vi "Actor Core.vi"(8 "error in":errorcluster, 11 "Instrument Finder in":refnum<class "Instrument Finder.lvclass">) -> (0 "error out":errorcluster, 3 "Actor out":refnum<class "Actor.lvclass">)   [LabVIEW 2014, in "SetUp VIs.lvlib" / "Instrument Finder.lvclass"]
doc: "(<B>Filename</B>: Actor Framework.lvlib:Actor.lvclass:Actor Core.vi)\n\nReceives messages to the actor, reacts to them, and initiates any error handling that may shut the actor down.\n\nDescendant classes may override this VI to append parallel tasks for the actor to complete while it handles messages. Overrides use the Call Parent Method node."
uses:
  Instrument Finder.lvclass
  <vilib>/ActorFramework/Actor/Actor.lvclass
  Controls/Instrument ID Object.ctl
  Generic Instrument/Generic Instrument.lvclass
  <vilib>/Instr/_visa.llb/VISA Find Search Mode.ctl
  <vilib>/ActorFramework/Actor/Actor.lvclass/Actor.ctl
  <vilib>/ActorFramework/Message Enqueuer/Message Enqueuer.lvclass/Message Enqueuer.ctl
  <vilib>/Utility/error.llb/DialogType.ctl
  <vilib>/ActorFramework/Report Error Msg/Report Error Msg.lvclass/Report Error Msg.ctl
  <vilib>/ActorFramework/Message Enqueuer/Message Priority.ctl
  Controller Messages/Write Instrument finder Done boolean to Ref Msg/Write Instrument finder Done boolean to Ref Msg.lvclass/Write Instrument finder Done boolean to Ref Msg.ctl
  <vilib>/ActorFramework/Stop Msg/Stop Msg.lvclass/Stop Msg.ctl
  Controller Messages/Write array of Instrument value to Ref Msg/Write array of Instrument value to Ref Msg.lvclass/Write array of Instrument value to Ref Msg.ctl
  <vilib>/ActorFramework/Message Enqueuer/Enqueue.vi
  <vilib>/ActorFramework/Message Enqueuer/Init from Existing Queue.vi
  <vilib>/ActorFramework/Message Enqueuer/Enqueue Critical.vi
  <vilib>/ActorFramework/Message Priority Queue/Priority Enqueue.vi
  <vilib>/ActorFramework/Report Error Msg/Report Error Msg.lvclass
  <vilib>/ActorFramework/Message Enqueuer/Message Enqueuer.lvclass
  Controller Messages/Write Instrument finder Done boolean to Ref Msg/Write Instrument finder Done boolean to Ref Msg.lvclass
  <vilib>/ActorFramework/Stop Msg/Stop Msg.lvclass
  Controller Messages/Write array of Instrument value to Ref Msg/Write array of Instrument value to Ref Msg.lvclass
  Subpanel Insertion/Subpanel Inserter.lvclass
  SetUp VIs.lvlib
panel:
  out "NaN/Path/Refnum?":bool
  out "done?":bool
  in  "Confirm":bool
  out "deleted portion 2":refnum<class "Generic Instrument.lvclass">
  out "Array":refnum<class "Generic Instrument.lvclass">[](array[class])
  out "error out 2":errorcluster
  out "deleted portion":T1
  out "# of time":i32
  out "selected instruments":T1[](array[typedef])
  out "index of element":i32
  out "data":T1
  out "find list":string[](array[string])
  out "i":i32
  out "Numeric Control":i32
  out "# of Instruments Found":i32
  in  "List of Instruments":T1[](array[typedef])
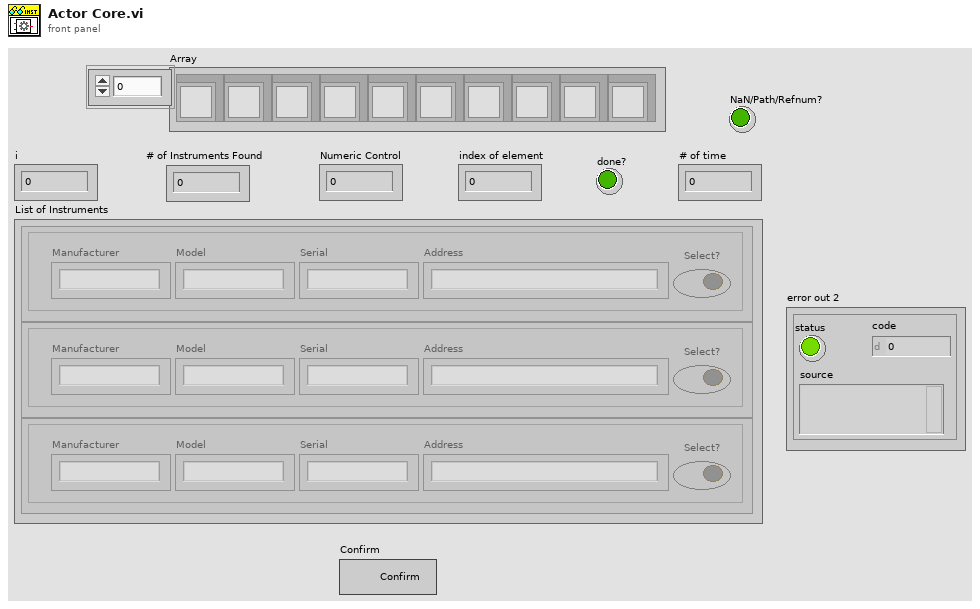
[diagram p1: front panel]
types:
  T1 = typedef "Instrument ID Object.ctl" = cluster{"Manufacturer":string, "Model":string, "Serial":string, "Address":string, "Select?":bool}
  T2 = cluster{"Manufacturer":string, "Model":string, "Serial":string, "Address":string, "Boolean":bool}[]
  T3 = typedef "VISA Find Search Mode.ctl" = u32
  T4 = typedef "DialogType.ctl" = u16
  T5 = typedef "Actor Framework.lvlib/Message Enqueuer.lvclass/Message Priority.ctl" = enum16{"Low", "Normal", "High"}
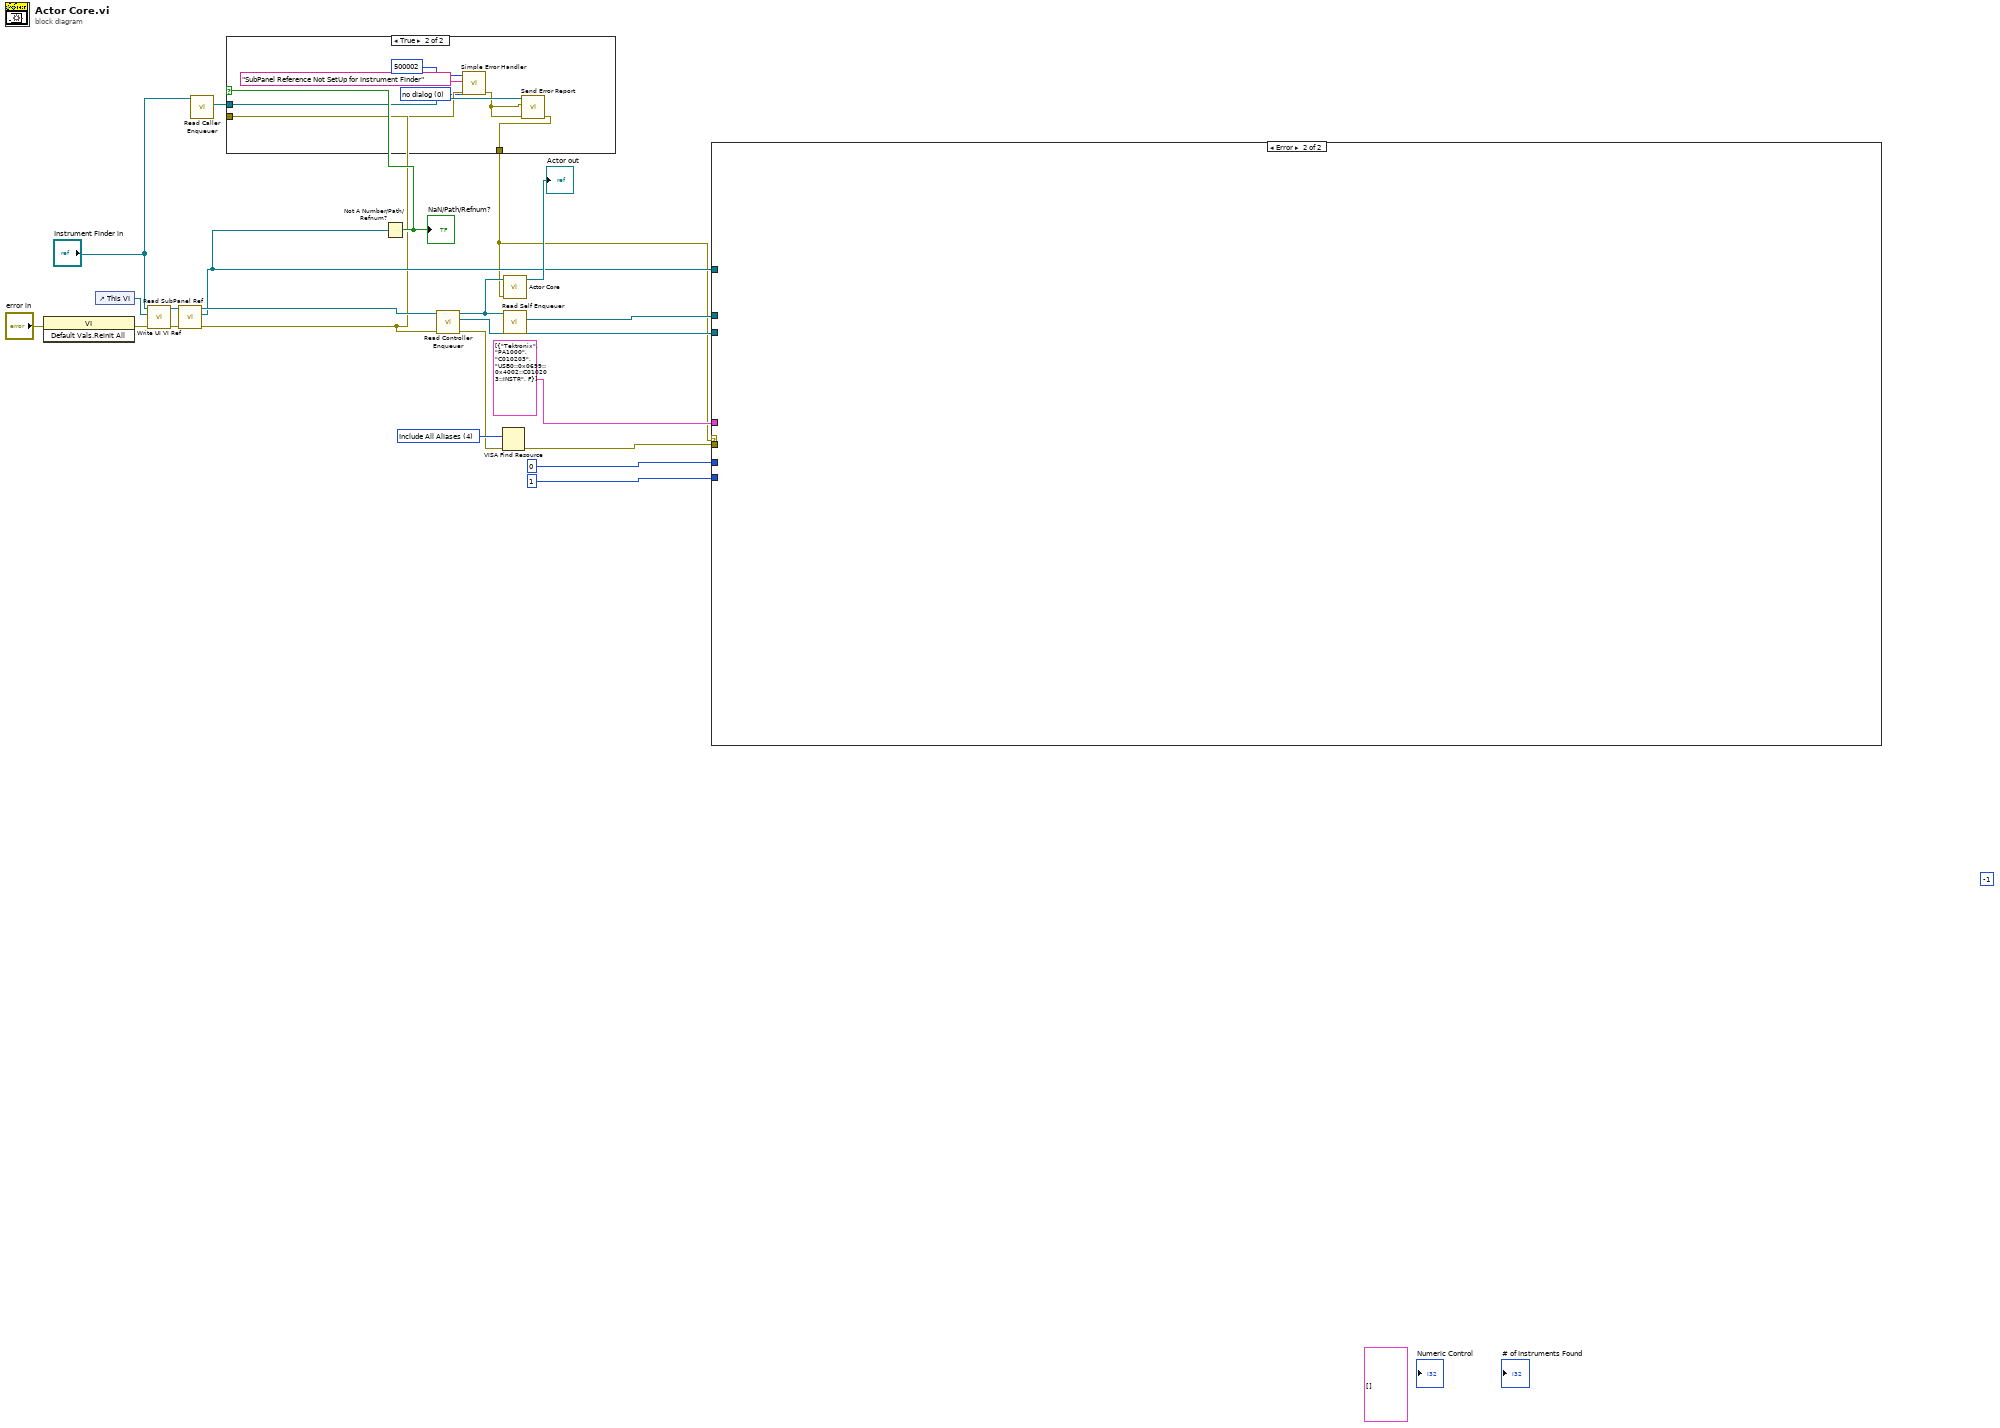
[diagram p0: block diagram]
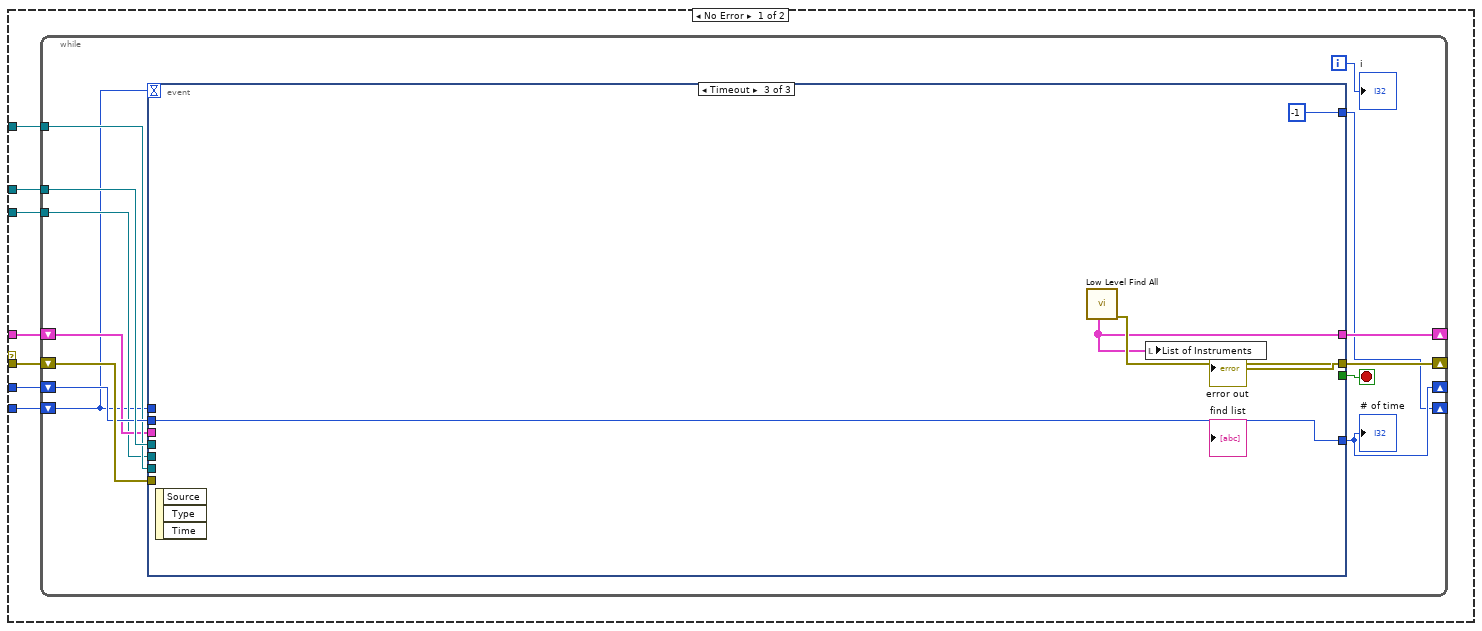
[diagram p2: hidden frame]
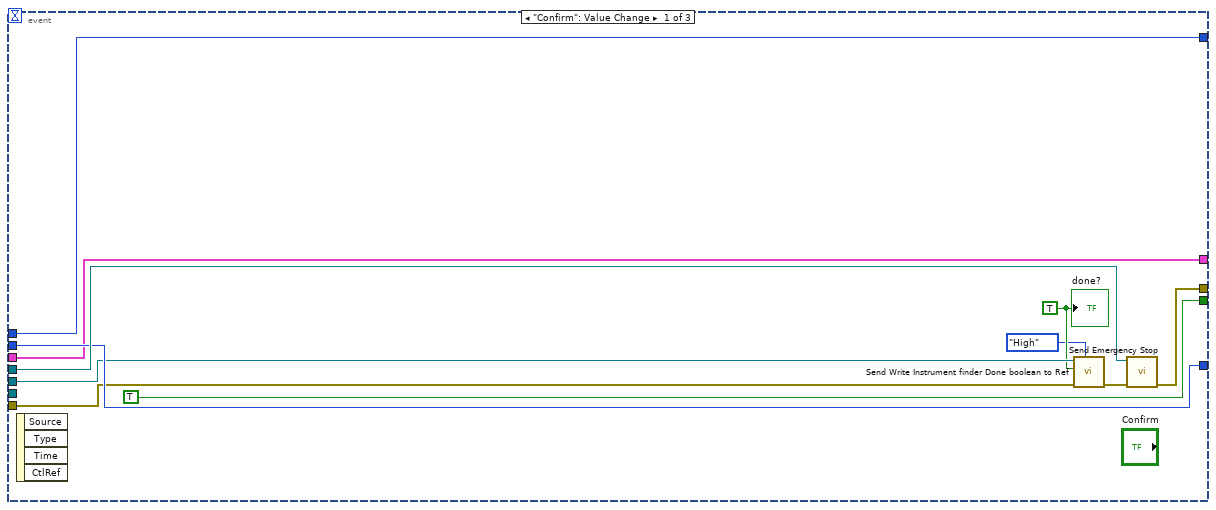
[diagram p3: hidden frame]
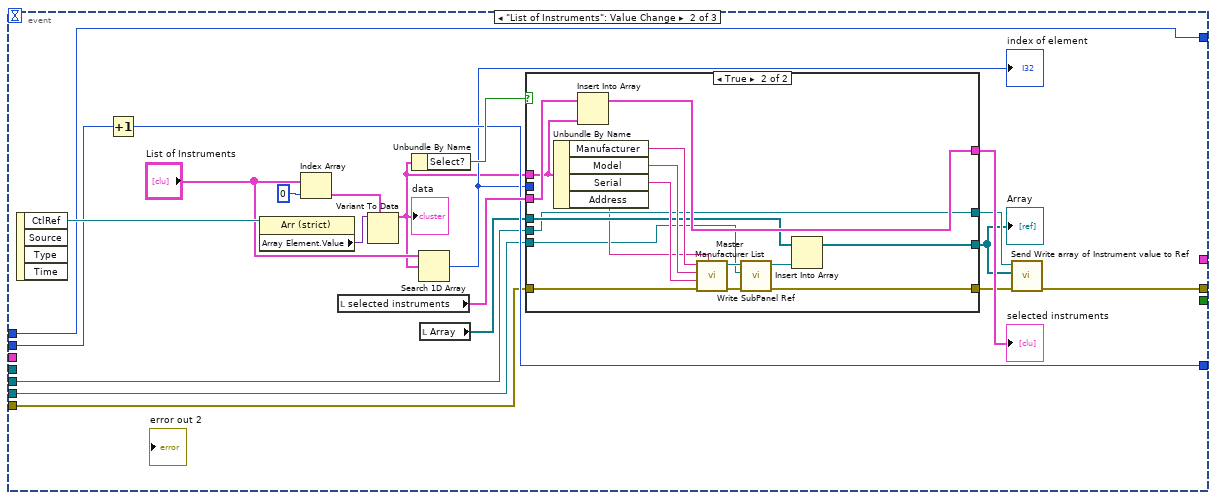
[diagram p4: hidden frame]
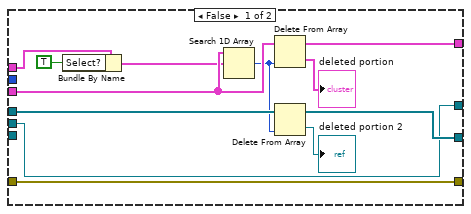
[diagram p5: hidden frame]
diagram:
  (unwired) -1
  (unwired) T1[] [] ("List of Instruments")
  w18 = T3 4 items=["Canonical Names Only"=0, "Aliases Only"=2, "Include Matching Aliases"=3, "Include All Aliases"=4] ("Search Mode")
  n1 = invoke class="VI" method="Default Vals.Reinit All"(error in="error in") -> (error out=w11:errorcluster)  [unwired: 2 in, 2 out]
  n2 = control-ref of="This VI"() -> (w12:refnum<vi>)
  n3 = call-dynamic "Write UI VI Ref.vi"("error in (no error)"=w11, "UI VI Ref"=w12, "Subpanel Inserter in"="Instrument Finder in") -> ("error out"=w13:errorcluster, "Subpanel Inserter out"=w14:refnum<class "Instrument Finder.lvclass">)  [unwired: 7 in]
  n4 = call-dynamic "Read SubPanel Ref.vi"("error in (no error)"=w13, "Subpanel Inserter in"=w14) -> ("error out"=w4:errorcluster, "SubPanel Ref"=w6:refnum<vi>, "Subpanel Inserter out"=w7:refnum<class "Instrument Finder.lvclass">)  [unwired: 7 in]
  n5 = call <vilib>:"Read Caller Enqueuer.vi"("Actor"="Instrument Finder in") -> ("Caller Enqueuer"=w2:refnum<class "Message Enqueuer.lvclass">)  [unwired: 10 in]
  n6 = Not A Number/Path/Refnum?(number/path/refnum=w6) -> (NaN/Path/Refnum?=w5:bool)
  "NaN/Path/Refnum?" <- w5
  n7 = case shown="True" w5 {
    tunnel: w4 -> [w23 w29]
    tunnel: w2 -> [_ w30]
    tunnel: [w23 w26] -> w1
    frame False {
    }
    frame True {
      w24 = T4 0 items=["no dialog", "OK message", "continue or stop message", "OK message + warnings", "continue/stop + warnings"] ("type of dialog (OK msg:1)")
      n8 = call <vilib>:"Simple Error Handler.vi"("error code (no error:0)"=500002 ("[error code] (0)"), "error source (\" \")"="SubPanel Reference Not SetUp for Instrument Finder" ("[error source] (\" \")"), "type of dialog (OK msg:1)"=w24, "error in (no error)"=w29) -> ("error out"=w27:errorcluster)  [unwired: 1 in, 4 out]
      n9 = call <vilib>:"Send Error Report.vi"("error in (no error)"=w27, "Error From Sender"=w27, "Message Enqueuer"=w30) -> ("error out"=w26:errorcluster)  [unwired: 8 in]
    }
  }
  n10 = call-dynamic "Read Controller Enqueuer.vi"("error in (no error)"=w4, "Instrument Finder in"=w7) -> ("error out"=w8:errorcluster, "Actor Framework:Message Enqueuer"=w10:refnum<class "Message Enqueuer.lvclass">, "Instrument Finder out"=w9:refnum<class "Instrument Finder.lvclass">)  [unwired: 7 in]
  n11 = VISA Find Resource(8:w8, 10:w18) -> (0:w19:errorcluster)  [unwired: 1 in, 2 out]
  n12 = call-parent "Actor Core.vi"("error in"=w1, "Actor in"=w9) -> ("Actor out"=→"Actor out":refnum<class "Actor.lvclass">)  [unwired: 8 in, 1 out]
  n13 = call <vilib>:"Read Self Enqueuer.vi"("Actor"=w9) -> ("Self Enqueuer"=w21:refnum<class "Message Enqueuer.lvclass">)  [unwired: 10 in]
  n14 = case shown="Error" w1 {
    tunnel: w21 -> [w38 _]
    tunnel: w19 -> [w37 _]
    tunnel: 1 -> [w36 _]
    tunnel: 0 ("index of element") -> [w34 _]
    tunnel: T2 [{"Manufacturer"="Tektronix", "Model"="PA1000", "Serial"="C010203", "Address"="USB0::0x0699::0x4002::C010203::INSTR", "Boolean"=FALSE}] ("List of Instruments") -> [w33 _]
    tunnel: w10 -> [w32 _]
    tunnel: w6 -> [w31 _]
    frame No Error {
      n15 = while {
        tunnel: w38 -> [w51]
        shift-right: [w49] -> w35
        shift-left: w37 -> [w50]
        shift-right: [w40] -> _
        shift-left: w36 -> [w39]
        shift-right: [w45] -> _
        shift-left: w34 -> [w46]
        tunnel: w31 -> [w44]
        shift-right: [w42] -> _
        shift-left: w33 -> [w43]
        tunnel: w32 -> [w41]
        i -> [w47]
        stop <- w48 stop-if-true
        n16 = event shown="[2] Timeout" {
          selector: _ -> [_ _ _]
          dyn-events: _ -> [_ _ _]
          timeout: w39 -> [_ _ _]
          tunnel: w51 -> [w62 _ _]
          tunnel: w50 -> [w54 w65 _]
          tunnel: [w60 w64 w115] -> w49
          tunnel: [TRUE _ _] -> w48
          tunnel: w46 -> [w59 w76 w114]
          tunnel: [w59 w75 w114] -> w45
          tunnel: w44 -> [_ w71 _]
          tunnel: w43 -> [w58 _ _]
          tunnel: [w58 _ w113] -> w42
          tunnel: w41 -> [w56 w69 _]
          tunnel: [w57 w68 -1] -> w40
          tunnel: w39 -> [w57 w68 _]
          event "Confirm": Value Change {
            w55 = TRUE ("Boolean")
            n17 = event-data() -> ()  [unwired: 1 in, 4 out]
            n18 = call "Send Write Instrument finder Done boolean to Ref.vi"("Message Priority (Normal)"=Message_Priority."High", "error in (no error)"=w54, "Boolean"=w55, "Message Enqueuer"=w56) -> ("error out"=w53:errorcluster)  [unwired: 6 in, 1 out]
            n19 = call <vilib>:"Send Emergency Stop.vi"("error in (no error)"=w53, "Message Enqueuer"=w62) -> ("error out"=w60:errorcluster)  [unwired: 9 in]
            "done?" <- w55
          }
          event "List of Instruments": Value Change {
            n20 = event-data() -> ("CtlRef"=w83:refnum<vi>)  [unwired: 1 in, 3 out]
            n21 = Increment(x=w76) -> (x+1=w75:i32)
            n22 = property class="Arr (strict)"(reference=w83) -> ("Array Element.Value"=w82:variant)  [unwired: 1 in, 2 out]
            n23 = Index Array(array="List of Instruments", index=0) -> (element=w80:T1)
            n24 = local read "selected instruments"() -> (w78:T1[])
            n25 = Variant To Data(type=w80, Variant=w82) -> (data=w73:T1)  [unwired: 1 in, 1 out]
            "data" <- w73
            n26 = Unbundle By Name(w73) -> ("Select?"=w77:bool)
            n27 = Search 1D Array(1D array="List of Instruments", element=w73) -> (index of element=w74:i32)  [unwired: 1 in]
            "index of element" <- w74
            n28 = local read "Array"() -> (w70:refnum<class "Generic Instrument.lvclass">[])
            n29 = case shown="True" w77 {
              tunnel: w78 -> [w94 w111]
              tunnel: [w95 w110] -> w72
              tunnel: w74 -> [_ _]
              tunnel: w73 -> [w92 w109]
              tunnel: w71 -> [_ w99]
              tunnel: w65 -> [w84 w105]
              tunnel: w70 -> [w89 w104]
              tunnel: [w87 w103] -> w66
              tunnel: w69 -> [w85 w102]
              tunnel: [w85 w102] -> w67
              tunnel: [w84 w96] -> w63
              frame False {
                n30 = Bundle By Name(cluster=w92, "Select?"=TRUE) -> (w91:T1)
                n31 = Search 1D Array(1D array=w94, element=w91) -> (index of element=w88:i32)  [unwired: 1 in]
                n32 = Delete From Array(array=w94, index=w88) -> (deleted portion=→"deleted portion":T1, array with subset deleted=w95:T1[])  [unwired: 1 in]
                n33 = Delete From Array(array=w89, index=w88) -> (deleted portion=→"deleted portion 2":refnum<class "Generic Instrument.lvclass">, array with subset deleted=w87:refnum<class "Generic Instrument.lvclass">[])  [unwired: 1 in]
              }
              frame True {
                n34 = Unbundle By Name(w109) -> ("Manufacturer"=w108:string, "Model"=w107:string, "Serial"=w106:string, "Address"=w101:string)
                n35 = Insert Into Array(array=w111, new element=w109) -> (w110:T1[])  [unwired: 1 in]
                n36 = call "Master Manufacturer List.vi"("VISA resource name"=w101, "error in"=w105, "Serial"=w106, "Model"=w107, "Manufacturer"=w108) -> ("error out"=w98:errorcluster, "Generic Instrument out"=w100:refnum<class "Generic Instrument.lvclass">)  [unwired: 5 in]
                n37 = call-dynamic "Write SubPanel Ref.vi"("error in (no error)"=w98, "SubPanel Ref"=w99, "Subpanel Inserter in"=w100) -> ("error out"=w96:errorcluster, "Subpanel Inserter out"=w97:refnum<class "Generic Instrument.lvclass">)  [unwired: 7 in]
                n38 = Insert Into Array(array=w104, new element=w97) -> (w103:refnum<class "Generic Instrument.lvclass">[])  [unwired: 1 in]
              }
            }
            "selected instruments" <- w72
            "Array" <- w66
            n39 = call "Send Write array of Instrument value to Ref.vi"("error in (no error)"=w63, "Array of Instruments"=w66, "Message Enqueuer"=w67) -> ("error out"=w64:errorcluster)  [unwired: 7 in, 1 out]
          }
          event Timeout {
            n40 = event-data() -> ()  [unwired: 1 in, 3 out]
            n41 = call "Low Level Find All.vi"() -> ("error out"=w115:errorcluster, "List of Instruments"=w113:T2)  [unwired: 5 in, 5 out]
            n42 = local write "List of Instruments"(w113) -> ()
          }
        }
        "# of time" <- w45
        "i" <- w47
      }
      "error out" <- w35
    }
    frame Error {
    }
  }
